vi "Wait for Result.vi"(11 "Async Authorization in":refnum<class "Async Authorization.lvclass">) -> (0 "error out":errorcluster, 1 "Result State":T1, 2 "Authorization":refnum<class "Authorization.lvclass">)   [LabVIEW 2020, in "OAuth2.lvlib" / "Async Authorization.lvclass"]
doc: "Blocks until the authorization flow completes either successfully or due to failure. If the user did not respond in time, Error 56 will be returned. If <b>Complete</b> result state is returned and there is no error then the authorization will be valid for use."
uses:
  Async Authorization.lvclass
  Authorization/Authorization.lvclass
  Async Auth State.ctl
  OAuth2.lvlib
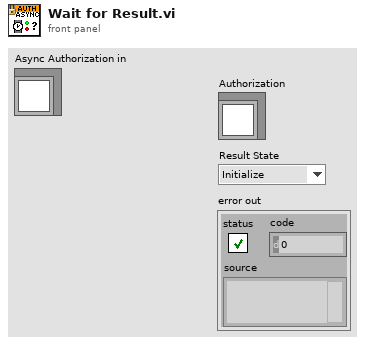
[diagram p1: front panel]
types:
  T1 = typedef "OAuth2.lvlib/Async Auth State.ctl" = enum16{"Initialize", "Request", "WaitAuth", "GetToken", "RefreshToken", "Complete", "Failed"}
  T2 = typedef "OAuth2.lvlib/Async Auth Result.ctl" = cluster{"Authorization":refnum<class "Authorization.lvclass">, "error":errorcluster}
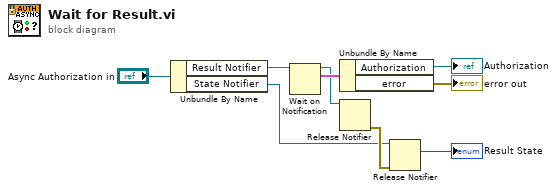
[diagram p0: block diagram]
diagram:
  n1 = Unbundle By Name("Async Authorization in") -> ("Result Notifier"=w8:refnum<notifier>, "State Notifier"=w2:refnum<notifier>)
  n2 = Wait on Notification(notifier=w8) -> (notifier out=w4:refnum<notifier>, notification=w7:T2)  [unwired: 3 in, 2 out]
  n3 = Unbundle By Name(w7) -> ("Authorization"=→"Authorization":refnum<class "Authorization.lvclass">, "error"=→"error out":errorcluster)
  n4 = Release Notifier(notifier=w4) -> (error out=w3:errorcluster)  [unwired: 2 in, 2 out]
  n5 = Release Notifier(notifier=w2, error in (no error)=w3) -> (last notification=→"Result State":T1)  [unwired: 1 in, 2 out]
